vi "Set AFG3252 pulse sequence.vi"(4 "Channel 2":dbl[](array[numeric]), 5 "Array size":dbl format="%#_13g", 6 "Channel 1":dbl[](array[numeric]), 7 "Gain (1 V)":dbl=1.0, 11 "VISA resource name":refnum<visa-resource-name>="USB0::0x0699::0x0345::C010498::INSTR") -> ()   [LabVIEW 2015]
doc: "Demonstrates how to configure then create an arbitrary waveform."
uses:
  Libraries/Tektronix AFG 3000 Series/Tektronix AFG 3000 Series.lvlib
panel:
  out "frequency":dbl format="%#_13g"
  # "10 MHz -> array size 200 -> 0.5 ns per 1 point\n1 MHz -> array size 2000 -> 0.5 ns per 1 point"
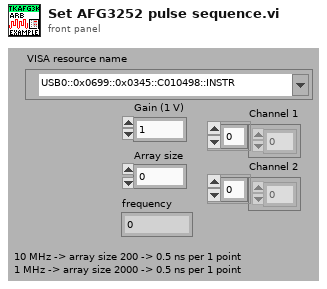
[diagram p1: front panel]
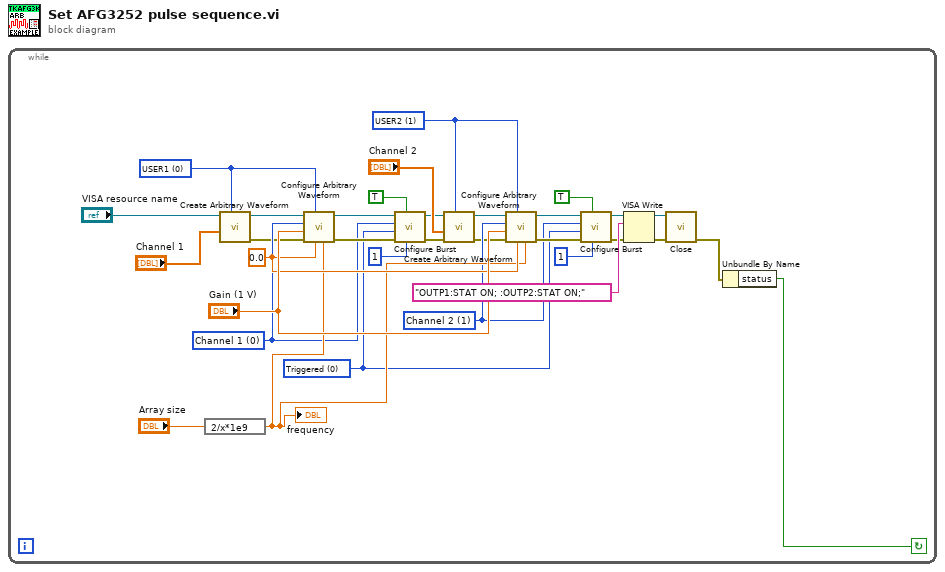
[diagram p0: block diagram]
diagram:
  n1 = while {
    stop <- w1 continue-if-true
    w15 = u16 0 items=["Triggered", "Gated"] ("Burst Mode (0: Triggered)")
    w31 = 0.0 ("DC Offset (0 V)")
    w17 = u16 0 items=["Channel 1", "Channel 2"] ("Channel (0: Channel 1)")
    w33 = u16 0 items=["USER1", "USER2", "USER3", "USER4"] ("Arbitrary Waveform Name (0: USER1)")
    w16 = u16 1 items=["Channel 1", "Channel 2"] ("Channel (0: Channel 1)")
    w30 = u16 1 items=["USER1", "USER2", "USER3", "USER4"] ("Arbitrary Waveform Name (0: USER1)")
    n2 = expression code="2/x*1e9"("Array size") -> (w28:dbl)
    "frequency" <- w28
    n3 = call "Create Arbitrary Waveform.vi"("Arbitrary Waveform Name (0: USER1)"=w33, "Arbitrary Waveform Data"="Channel 1", "VISA resource name"="VISA resource name") -> ("error out"=w10:errorcluster, "VISA resource name out"=w11:refnum<visa-resource-name>)  [unwired: 7 in]
    n4 = call "Configure Arbitrary Waveform.vi"("Frequency (1000 Hz)"=w28, "DC Offset (0 V)"=w31, "Arbitrary Waveform Name (0: USER1)"=w33, "error in (no error)"=w10, "Gain (1 V)"="Gain (1 V)", "Channel (0: Channel 1)"=w17, "VISA resource name"=w11) -> ("error out"=w26:errorcluster, "VISA resource name out"=w27:refnum<visa-resource-name>)  [unwired: 3 in]
    n5 = call "Configure Burst.vi"("Burst Count (5)"=1, "Enable Burst (T: Enable)"=TRUE, "error in (no error)"=w26, "Burst Mode (0: Triggered)"=w15, "Channel (0: Channel 1)"=w17, "VISA resource name"=w27) -> ("error out"=w8:errorcluster, "VISA resource name out"=w9:refnum<visa-resource-name>)  [unwired: 4 in]
    n6 = call "Create Arbitrary Waveform.vi"("Arbitrary Waveform Name (0: USER1)"=w30, "error in (no error)"=w8, "Arbitrary Waveform Data"="Channel 2", "VISA resource name"=w9) -> ("error out"=w12:errorcluster, "VISA resource name out"=w13:refnum<visa-resource-name>)  [unwired: 6 in]
    n7 = call "Configure Arbitrary Waveform.vi"("Frequency (1000 Hz)"=w28, "DC Offset (0 V)"=w31, "Arbitrary Waveform Name (0: USER1)"=w30, "error in (no error)"=w12, "Gain (1 V)"="Gain (1 V)", "Channel (0: Channel 1)"=w16, "VISA resource name"=w13) -> ("error out"=w24:errorcluster, "VISA resource name out"=w25:refnum<visa-resource-name>)  [unwired: 3 in]
    n8 = call "Configure Burst.vi"("Burst Count (5)"=1, "Enable Burst (T: Enable)"=TRUE, "error in (no error)"=w24, "Burst Mode (0: Triggered)"=w15, "Channel (0: Channel 1)"=w16, "VISA resource name"=w25) -> ("error out"=w5:errorcluster, "VISA resource name out"=w6:refnum<visa-resource-name>)  [unwired: 4 in]
    n9 = VISA Write(VISA resource name=w6, write buffer="OUTP1:STAT ON; :OUTP2:STAT ON;", error in (no error)=w5) -> (VISA resource name out=w4:refnum<visa-resource-name>, error out=w3:errorcluster)  [unwired: 1 out]
    n10 = call "Close.vi"("error in (no error)"=w3, "VISA resource name"=w4) -> ("error out"=w2:errorcluster)  [unwired: 9 in]
    n11 = Unbundle By Name(w2) -> ("status"=w1:bool)
  }
